vi "Get Label Ref and Caption Ref From Control(冲突时的文件备份2013-05-03 10-35-22).vi"(8 "错误输入（无错误）":errorcluster, 11 "Ctl Ref In":refnum<vi>) -> (0 "错误输出":errorcluster, 1 "Caption Ref":refnum<vi>, 2 "Label Ref":refnum<vi>, 3 "Ctl Ref Out":refnum<vi>, 4 "Caption Created":bool)   [LabVIEW 2012, in "CtrlRef.lvlib"]
uses:
  CtrlRef.lvlib
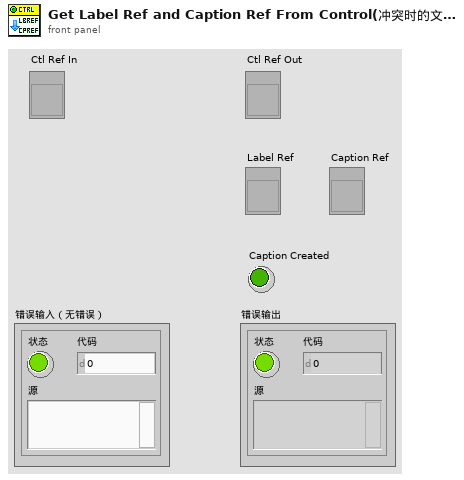
[diagram p1: front panel]
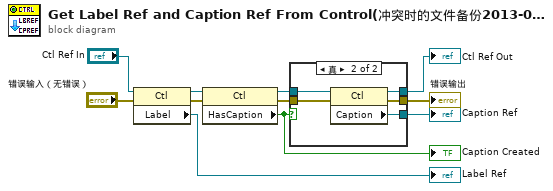
[diagram p0: block diagram]
diagram:
  n1 = property class="Ctl"(reference="Ctl Ref In", error in="错误输入（无错误）") -> (reference out=w7:refnum<vi>, error out=w8:errorcluster, "Label"=→"Label Ref":refnum<vi>)
  n2 = property class="Ctl"(reference=w7, error in=w8) -> (reference out=w2:refnum<vi>, error out=w4:errorcluster, "HasCaption"=w5:bool)
  "Caption Created" <- w5
  n3 = case shown="真" w5 {
    tunnel: [_ w18] -> w6
    tunnel: w4 -> [w12 w17]
    tunnel: [w12 w16] -> w3
    tunnel: w2 -> [w13 w15]
    tunnel: [w13 w14] -> w1
    frame False {
    }
    frame True {
      n4 = property class="Ctl"(reference=w15, error in=w17) -> (reference out=w14:refnum<vi>, error out=w16:errorcluster, "Caption"=w18:refnum<vi>)
    }
  }
  "错误输出" <- w3
  "Ctl Ref Out" <- w1
  "Caption Ref" <- w6
